vi "write_read_comand.vi"() -> ()   [LabVIEW 2022 SP3]
panel:
  in  "byte8":u8 format="%x"
  in  "byte7":u8 format="%x"
  in  "byte6":u8 format="%x"
  in  "byte5":u8 format="%x"
  in  "byte4":u8=246 format="%x"
  in  "byte3":u8=128 format="%x"
  in  "Other_byte":u8=254 format="%x"
  in  "First_byte":u8=178 format="%x"
  out "InputReport1":u8[](array[numeric]) format="%x"
  out "Output Report":u8[](array[numeric])
  out "Input Report":u8[](array[numeric])
  # "FF - output 1, FE - output 2"
  # "voltage"
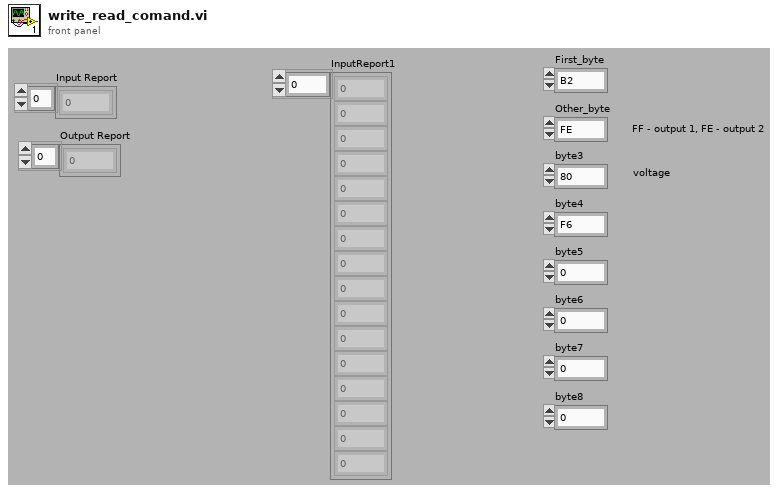
[diagram p1: front panel]
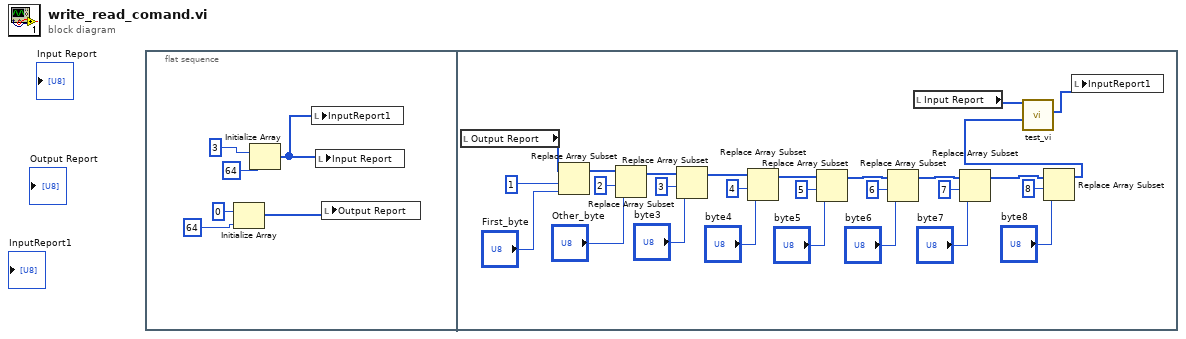
[diagram p0: block diagram]
diagram:
  n1 = flat-sequence {
    frame #0 {
      n2 = Initialize Array(u8 0 ("element"), 64 ("dimension size")) -> (w2:u8[])
      n3 = Initialize Array(u8 3 ("element"), 64 ("dimension size")) -> (w1:u8[])
      n4 = local write "InputReport1"(w1) -> ()
      n5 = local write "Input Report"(w1) -> ()
      n6 = local write "Output Report"(w2) -> ()
    }
    frame #1 {
      n7 = local read "Output Report"() -> (w32:u8[])
      n8 = Replace Array Subset(array=w32, new element="First_byte", index=1) -> (w28:u8[])
      n9 = Replace Array Subset(array=w28, new element="Other_byte", index=2) -> (w25:u8[])
      n10 = Replace Array Subset(array=w25, new element="byte3", index=3) -> (w12:u8[])
      n11 = Replace Array Subset(array=w12, new element="byte4", index=4) -> (w11:u8[])
      n12 = Replace Array Subset(array=w11, new element="byte5", index=5) -> (w10:u8[])
      n13 = Replace Array Subset(array=w10, new element="byte6", index=6) -> (w9:u8[])
      n14 = local read "Input Report"() -> (w31:u8[])
      n15 = Replace Array Subset(array=w9, new element="byte7", index=7) -> (w8:u8[])
      n16 = Replace Array Subset(array=w8, new element="byte8", index=8) -> (w7:u8[])
      n17 = call "test_vi.vi"("OutputReport_in"=w7, "InputReport_in"=w31) -> ("InputReport_out"=w30:u8[])  [unwired: 2 in, 3 out]
      n18 = local write "InputReport1"(w30) -> ()
    }
  }
